vi "SortidaDigitalUSB.vi"(2 "stop":refnum<vi>, 4 "SortidesDigitals":refnum<vi>) -> ()   [LabVIEW 2017]
uses:
  <vilib>/DAQmx/write.llb/DAQmx Write (Digital 1D Bool NChan 1Samp 1Line).vi
  <vilib>/DAQmx/miscellaneous.llb/DAQmx Fill In Error Info.vi
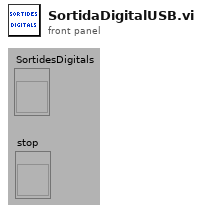
[diagram p1: front panel]
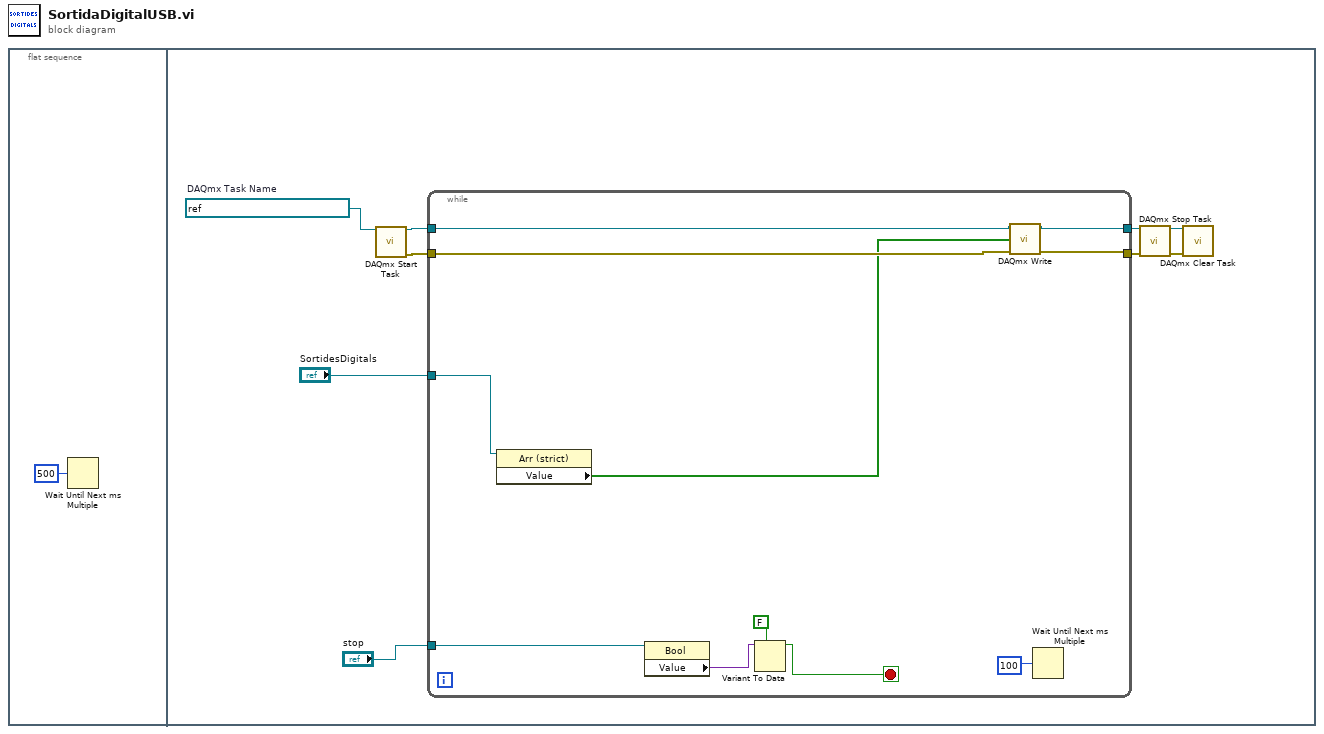
[diagram p0: block diagram]
diagram:
  n1 = flat-sequence {
    frame #0 {
      n2 = Wait Until Next ms Multiple(millisecond multiple=u32 500) -> ()  [unwired: 1 out]
    }
    frame #1 {
      w5 = refnum<k21> "TallGuants_USBDigitalOut"  # DAQmx Task Name
      n3 = call <vilib>:"DAQmx Start Task.vi"("task/channels in"=w5) -> ("task out"=w10:refnum<k21>, "error out"=w8:errorcluster)  [unwired: 13 in]
      n4 = while {
        tunnel: w10 -> [w16]
        tunnel: [w14] -> w9
        tunnel: w8 -> [w15]
        tunnel: [w13] -> w7
        tunnel: "stop" -> [w20]
        tunnel: "SortidesDigitals" -> [w11]
        stop <- w17 stop-if-true
        n5 = property class="Arr (strict)"(reference=w11) -> ("Value"=w12:bool[])  [unwired: 1 in, 2 out]
        n6 = property class="Bool"(reference=w20) -> ("Value"=w19:variant)  [unwired: 1 in, 2 out]
        n7 = Variant To Data(type=FALSE ("stop"), Variant=w19) -> (data=w17:bool)  [unwired: 1 in, 1 out]
        n8 = call-poly <vilib>:"DAQmx Write.vi"("task/channels in"=w16, "data"=w12, "error in"=w15) -> ("task out"=w14:refnum<k21>, "error out"=w13:errorcluster)  [unwired: 10 in, 1 out]
        n9 = Wait Until Next ms Multiple(millisecond multiple=u32 100) -> ()  [unwired: 1 out]
      }
      n10 = call <vilib>:"DAQmx Stop Task.vi"("task/channels in"=w9, "error in"=w7) -> ("task out"=w3:refnum<k21>, "error out"=w2:errorcluster)  [unwired: 12 in]
      n11 = call <vilib>:"DAQmx Clear Task.vi"("task in"=w3, "error in"=w2) -> ()  [unwired: 13 in, 1 out]
    }
  }
